vi "PC Main.vi"() -> ()   [LabVIEW 2021]
uses:
  Typedefs/Q FGV State Command.ctl
  Typedefs/Q Message Data.ctl
  <vilib>/event_ctls.llb/eventvkey.ctl
  <vilib>/Utility/error.llb/Error Cluster From Error Code.vi
  <vilib>/ErrorRing/Error Ring.xnode
panel:
  in  "Tab Control Application":enum32{"Home", "Measuring Panel"}(tab)
  in  "Connect Button":bool
  in  "NI-sbRIO-9651 IP address":string="10.8.5.60"
  in  "New Measurement Button":bool
  in  "Contact Button 1":bool
  in  "Close Button 1":bool
  in  "System Information Button 1":bool
  in  "Contact Button 2":bool
  in  "Close Button 2":bool
  in  "System Information Button 2":bool
  in  "Tab Control sbRIO":enum32{"Page 1"}(tab)
  in  "Reset Button":bool
  in  "Disconnect Button":bool
  # "3-Phase Power Meter \non the NI9651 circuit"
  # "NI-sbRIO-9651 Control"
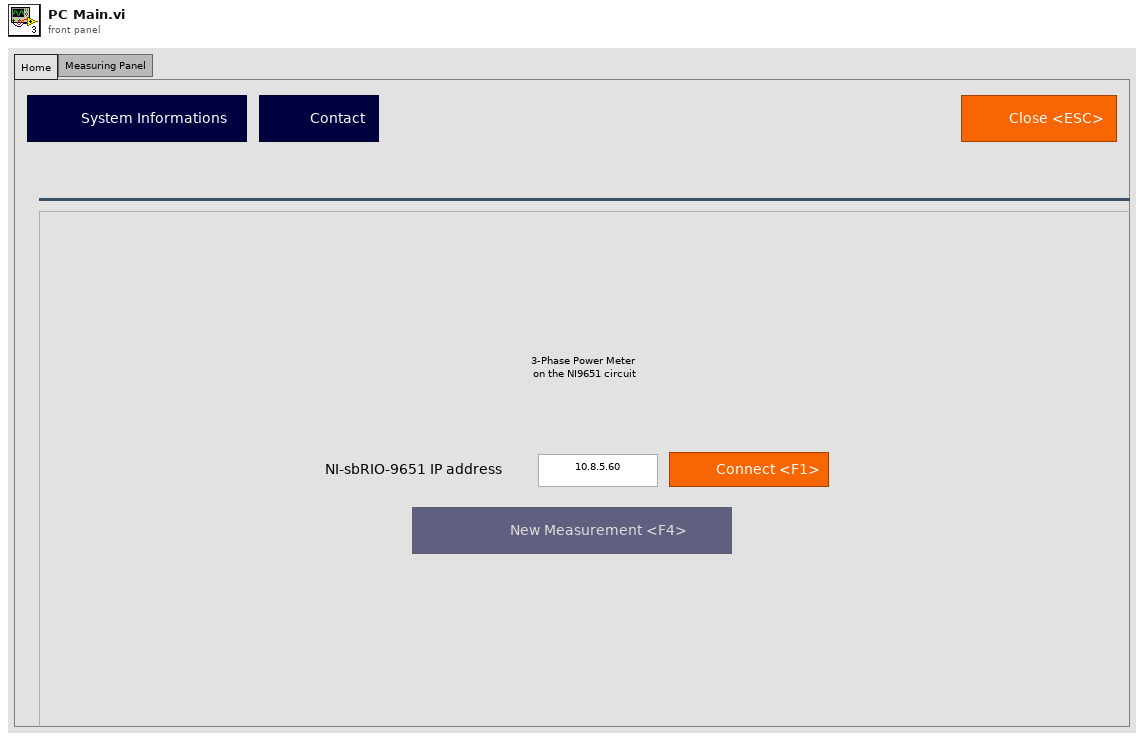
[diagram p1: front panel]
types:
  T1 = typedef "Q FGV State Command.ctl" = enum16{"Initialize", "Get", "Release"}
  T2 = typedef "Q Message Data.ctl" = cluster{"State Command":string, "Data":variant}
  T3 = enum8{"Enabled", "Disabled", "Disabled and Grayed Out"}
  T4 = typedef "eventvkey.ctl" = enum16{"ASCII", "Enter", "Return", "Shift", "Ctrl", "Alt", "Cmd", "Opt", "Caps", "NumLock", "Clear", "Break", "Up", "Down", "Left", "Right", "Insert", "Delete", "Home", "End", "PageUp", "PageDown", "Escape", "Help", "Pause", "ScrollLock", "F1", "F2", "F3", "F4", "F5", "F6", "F7", "F8", "F9", "F10", "F11", "F12", "F13", "F14", "F15", "F16", "F17", "F18", "F19", "F20", "F21", "F22", "F23", "F24", "Play", "VolumeUp", "VolumeDown", "Mute", "Two Byte Char"}
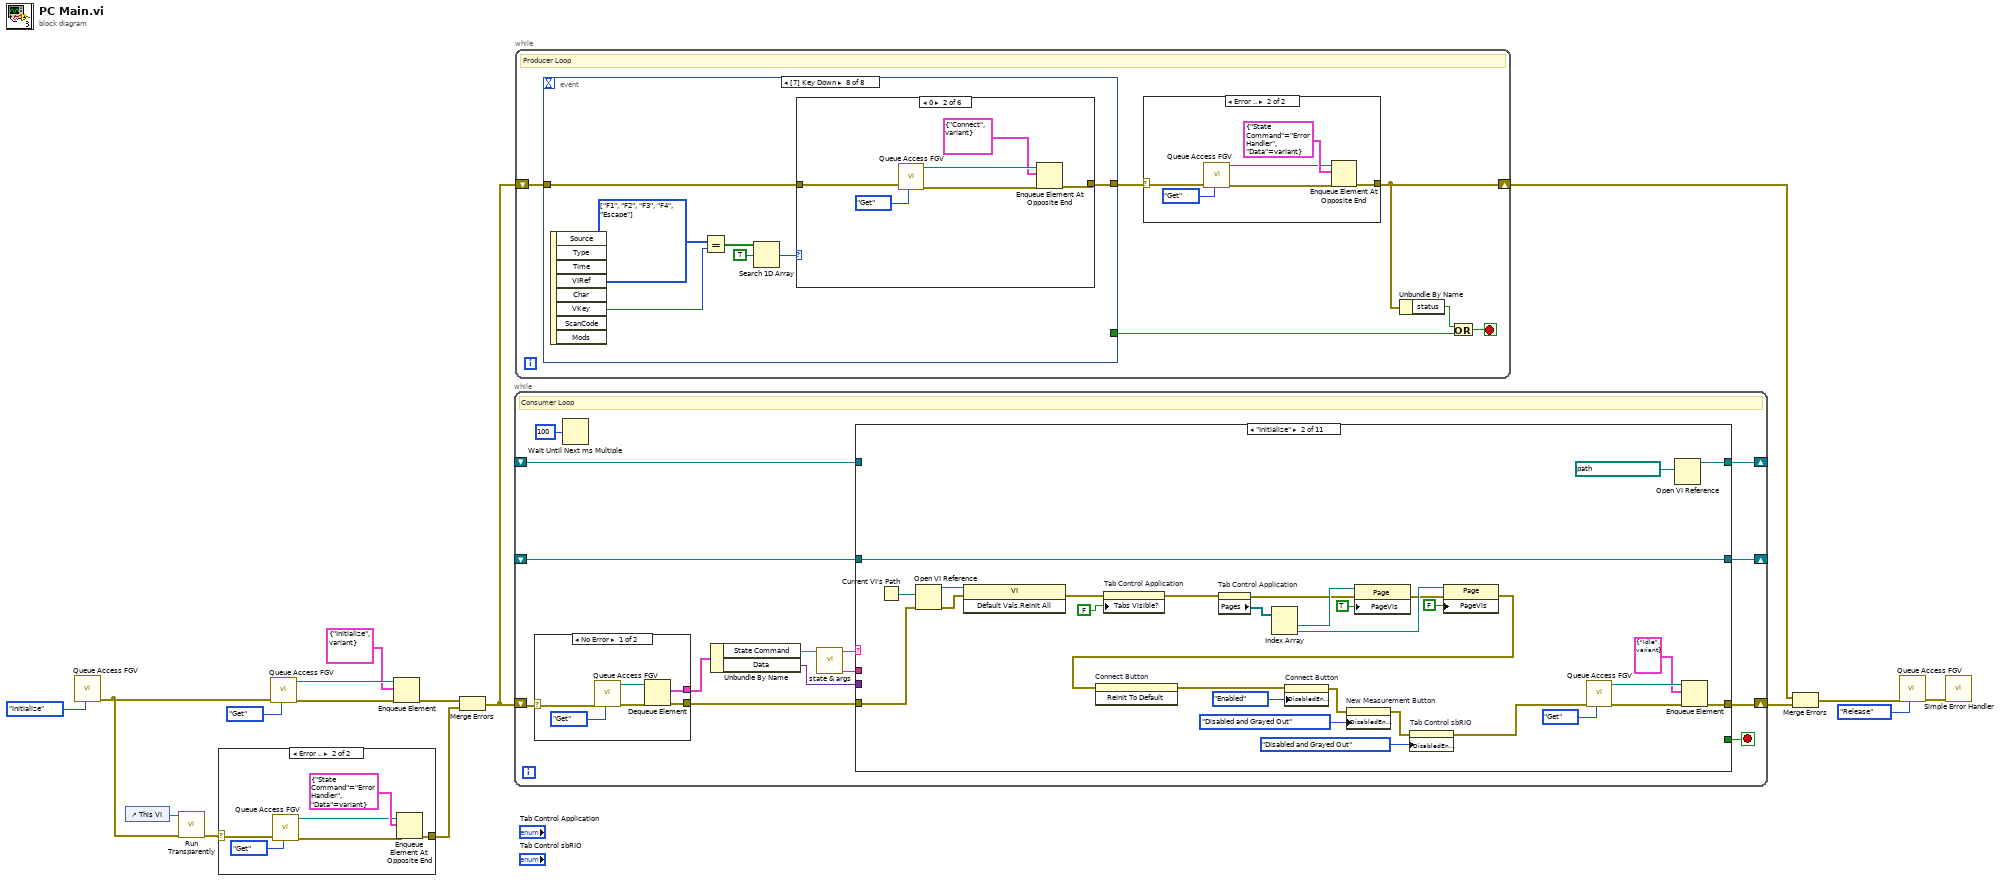
[diagram p0: block diagram]
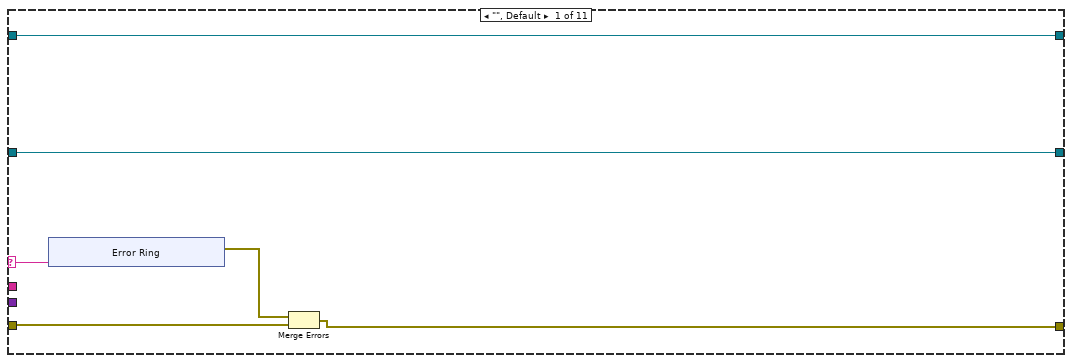
[diagram p3: hidden frame]
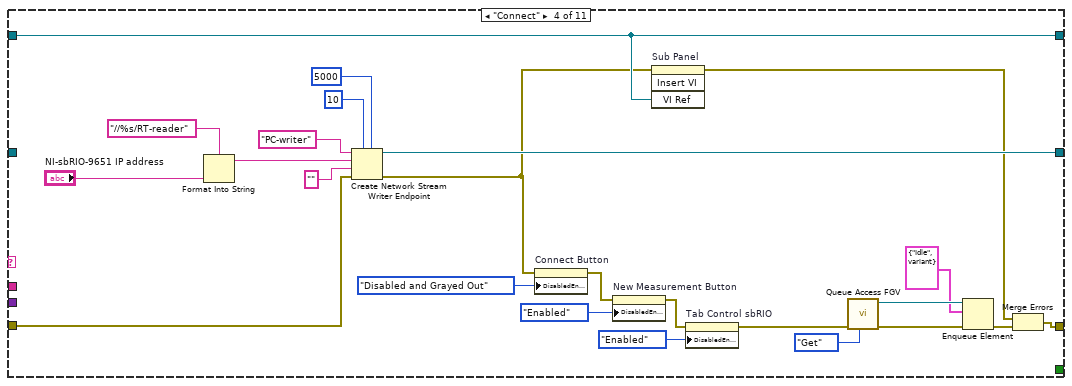
[diagram p5: hidden frame]
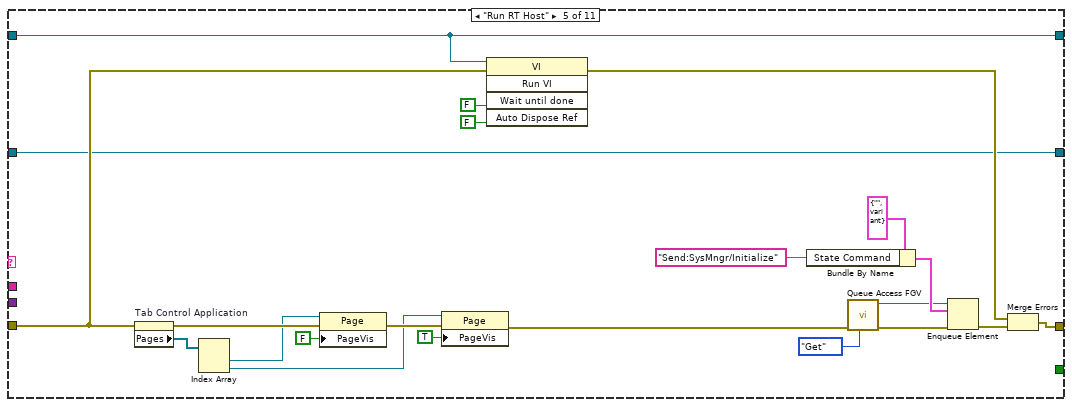
[diagram p6: hidden frame]
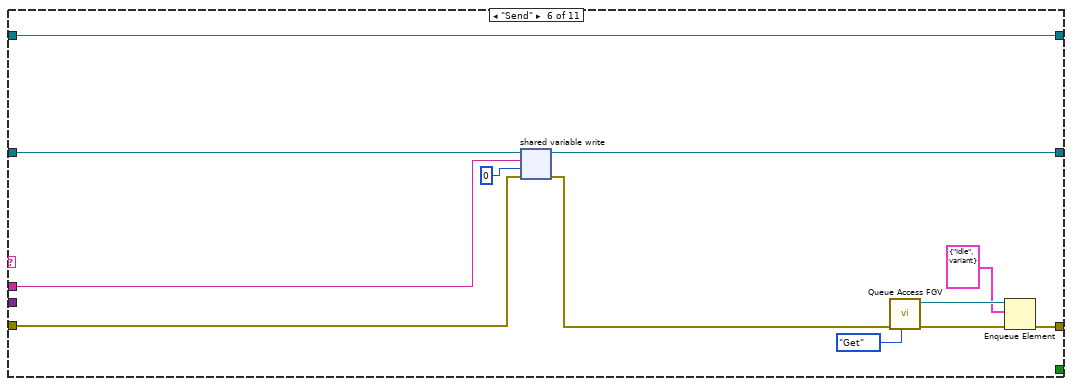
[diagram p7: hidden frame]
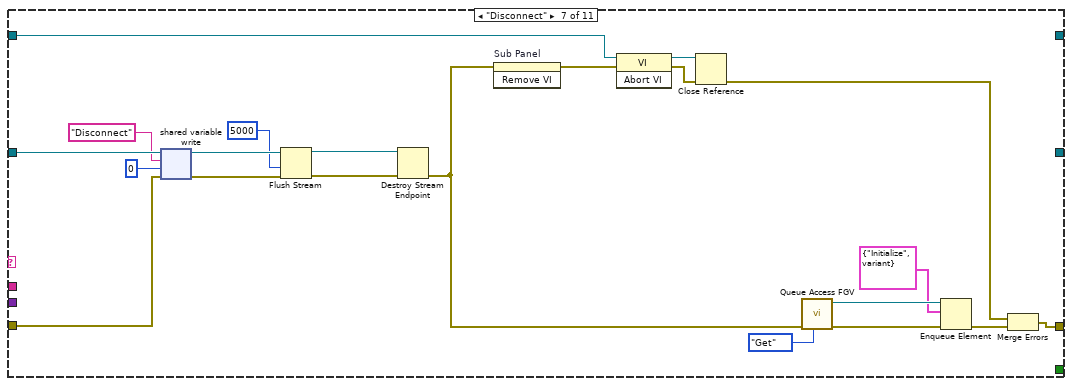
[diagram p8: hidden frame]
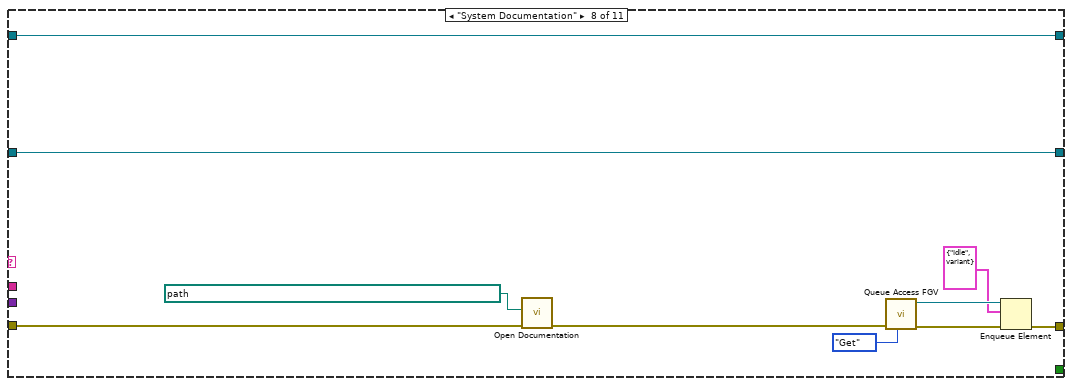
[diagram p9: hidden frame]
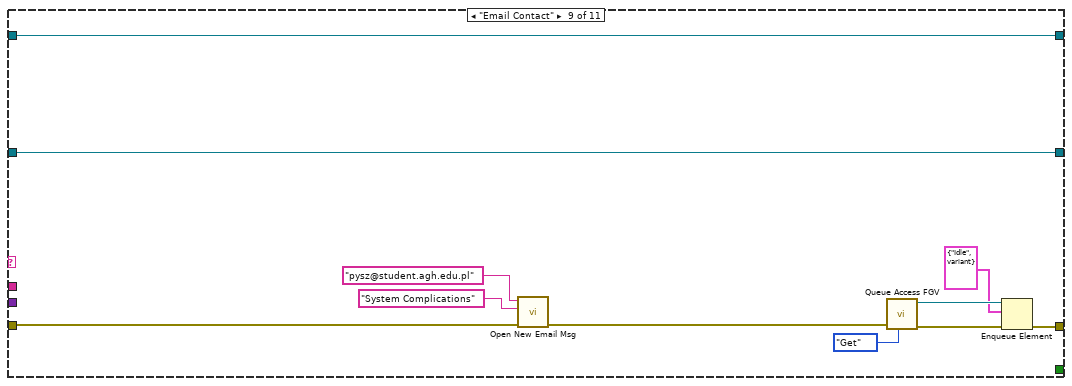
[diagram p10: hidden frame]
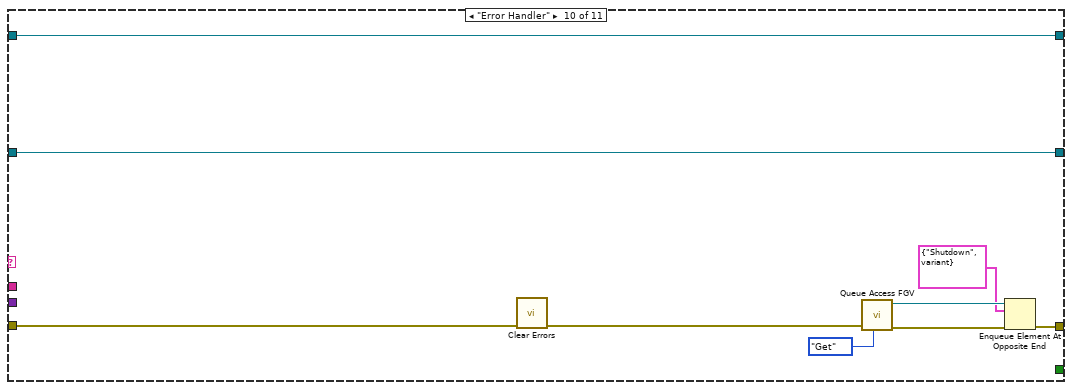
[diagram p11: hidden frame]
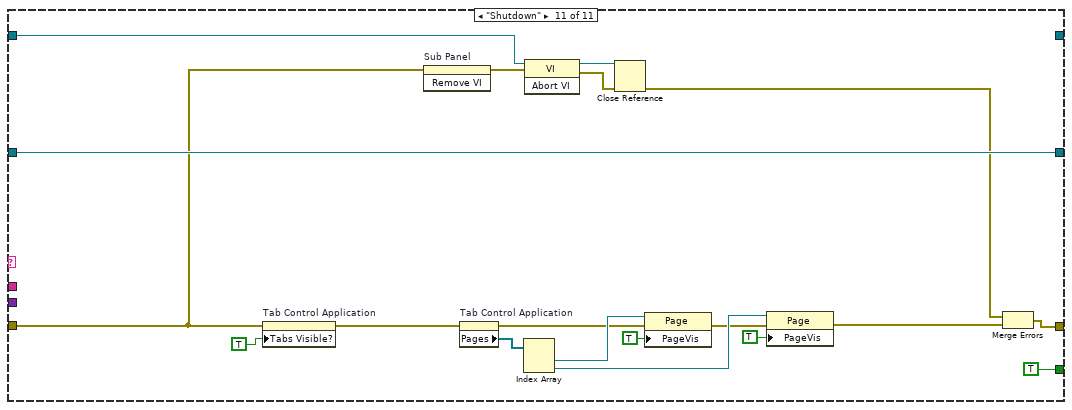
[diagram p12: hidden frame]
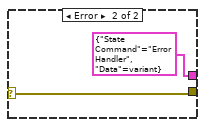
[diagram p13: hidden frame]
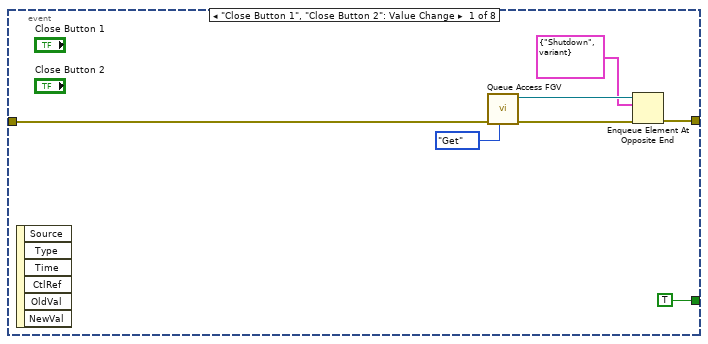
[diagram p14: hidden frame]
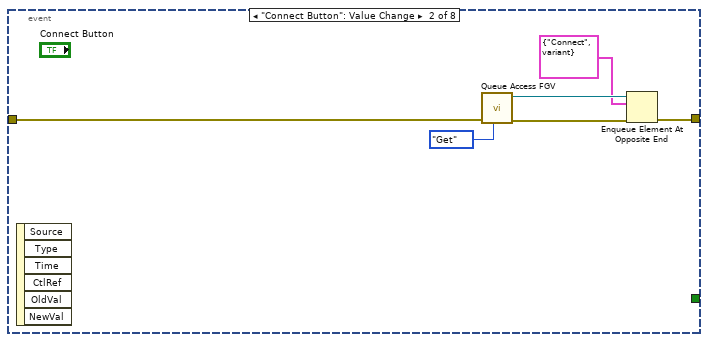
[diagram p15: hidden frame]
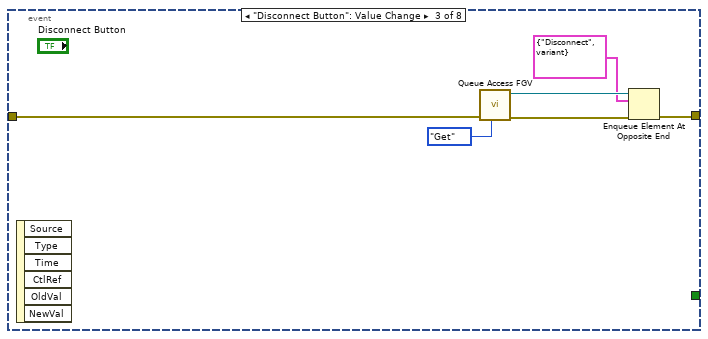
[diagram p16: hidden frame]
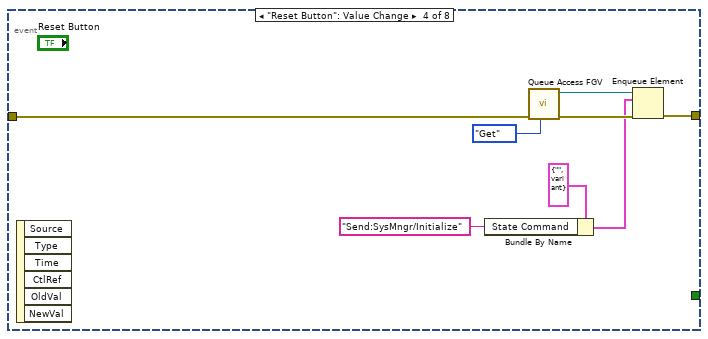
[diagram p17: hidden frame]
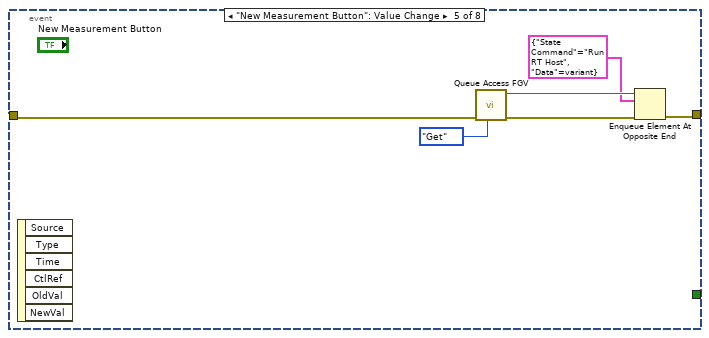
[diagram p18: hidden frame]
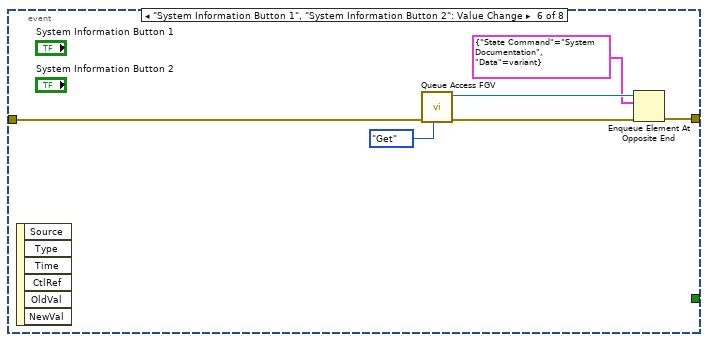
[diagram p19: hidden frame]
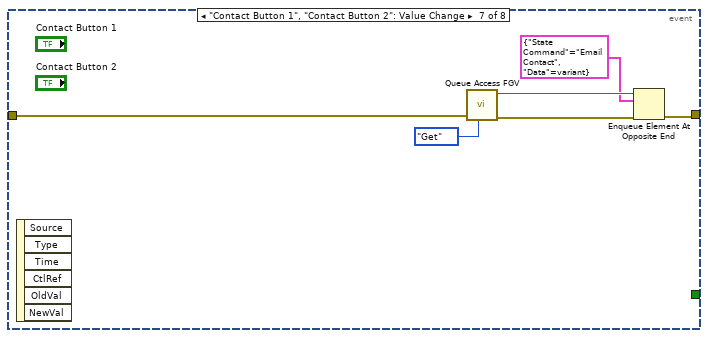
[diagram p20: hidden frame]
diagram:
  n1 = call "Queue Access FGV.vi"("FGV State Command"=Q_FGV_State_Command."Initialize") -> ("error out"=w5:errorcluster)  [unwired: 9 in, 1 out]
  n2 = control-ref of="This VI"() -> (w3:refnum<vi>)
  n3 = call "Run Transparently.vi"("error in (no error)"=w5, "This VI"=w3) -> ("error out"=w9:errorcluster)  [unwired: 9 in]
  n4 = case shown="Error .." w9 {
    selector: w9 -> [w17 w23]
    tunnel: [w17 w21] -> w6
    frame No Error {
    }
    frame Error {
      n5 = call "Queue Access FGV.vi"("FGV State Command"=Q_FGV_State_Command."Get", "error in (no error)"=w23) -> ("error out"=w22:errorcluster, "queue out"=w18:refnum<queue>)  [unwired: 8 in]
      n6 = Enqueue Element At Opposite End(queue=w18, element=T2 {"State Command"="Error Handler", "Data"=variant}, error in (no error)=w22) -> (error out=w21:errorcluster)  [unwired: 1 in, 2 out]
    }
  }
  n7 = call "Queue Access FGV.vi"("FGV State Command"=Q_FGV_State_Command."Get", "error in (no error)"=w5) -> ("error out"=w14:errorcluster, "queue out"=w15:refnum<queue>)  [unwired: 8 in]
  n8 = Enqueue Element(queue=w15, element=T2 {"State Command"="Initialize", "Data"=variant}, error in (no error)=w14) -> (error out=w7:errorcluster)  [unwired: 1 in, 2 out]
  n9 = Merge Errors(w7, w6) -> (w8:errorcluster)
  n10 = while {
    shift-right: [w27] -> _
    shift-left: _ -> [w28]
    shift-right: [w26] -> _
    shift-left: _ -> [w25]
    shift-right: [w24] -> w2
    shift-left: w8 -> [w37]
    stop <- w29 stop-if-true
    # "Consumer Loop"
    n11 = case shown="No Error" w37 {
      selector: w37 -> [w216 w219]
      tunnel: [w213 w219] -> w35
      tunnel: [w212 T2 {"State Command"="Error Handler", "Data"=variant} ("element")] -> w36
      frame No Error {
        n12 = call "Queue Access FGV.vi"("FGV State Command"=Q_FGV_State_Command."Get", "error in (no error)"=w216) -> ("error out"=w214:errorcluster, "queue out"=w217:refnum<queue>)  [unwired: 8 in]
        n13 = Dequeue Element(queue=w217, error in (no error)=w214) -> (element=w212:T2, error out=w213:errorcluster)  [unwired: 1 in, 2 out]
      }
      frame Error {
      }
    }
    n14 = Wait Until Next ms Multiple(millisecond multiple=u32 100) -> ()  [unwired: 1 out]
    n15 = Unbundle By Name(w36) -> ("State Command"=w34:string, "Data"=w31:variant)
    n16 = call "state & args.vi"("state:args"=w34) -> ("args"=w32:string, "state"=w33:string)  [unwired: 9 in]
    n17 = case shown="\"Initialize\"" w33 {
      selector: w33 -> [w43 _ _ _ _ _ _ _ _ _ _]
      tunnel: w35 -> [w41 w67 w83 w88 w112 w141 w155 w167 w178 w192 w196]
      tunnel: [w40 w73 w83 w85 w110 w133 w143 w168 w179 w186 w194] -> w24
      tunnel: w32 -> [_ _ _ _ _ w138 _ _ _ _ _]
      tunnel: w31 -> [_ _ _ _ _ _ _ _ _ _ _]
      tunnel: [_ _ _ _ _ _ _ _ _ _ TRUE] -> w29
      tunnel: w28 -> [w39 w51 w82 _ w108 w140 w158 w164 w173 w185 w210]
      tunnel: [w39 w51 w82 w94 w108 w139 _ w164 w173 w185 w210] -> w27
      tunnel: [w38 w52 w81 w89 w113 w131 _ w163 w174 w184 _] -> w26
      tunnel: w25 -> [w38 _ w81 w89 w113 w131 w148 w163 w174 w184 w200]
      frame "", Default {
        n18 = xnode "Error Ring"("parameter 0"=w43) -> ("error out"=w42:errorcluster)
        n19 = Merge Errors(w42, w41) -> (w40:errorcluster)
      }
      frame "Initialize" {
        n20 = Current VI's Path() -> (path=w80:path)
        n21 = Open VI Reference(vi path=w80, error in (no error)=w67) -> (vi reference=w79:refnum<vi>, error out=w78:errorcluster)  [unwired: 4 in]
        n22 = invoke class="VI" method="Default Vals.Reinit All"(reference=w79, error in=w78) -> (error out=w57:errorcluster)  [unwired: 1 in, 2 out]
        n23 = property on="Tab Control Application" class="TabCtl (strict)"(error in=w57, "Tabs Visible?"=FALSE) -> (error out=w66:errorcluster)  [unwired: 1 in, 1 out]
        n24 = property on="Tab Control Application" class="TabCtl (strict)"(error in=w66) -> (error out=w62:errorcluster, "Pages"=w61:refnum<vi>[])  [unwired: 1 in, 1 out]
        n25 = Index Array(array=w61) -> (element #1=w63:refnum<vi>, element #2=w65:refnum<vi>)  [unwired: 2 in]
        n26 = property class="Page"(reference=w63, error in=w62, "PageVis"=TRUE ("Page Visible")) -> (error out=w64:errorcluster)  [unwired: 1 out]
        n27 = property class="Page"(reference=w65, error in=w64, "PageVis"=FALSE ("Page Visible")) -> (error out=w55:errorcluster)  [unwired: 1 out]
        n28 = invoke on="Connect Button" class="Bool" method="Reinit To Default"(error in=w55) -> (error out=w56:errorcluster)  [unwired: 2 in, 2 out]
        n29 = property on="Connect Button" class="Bool"(error in=w56, "DisabledEnum"=T3."Enabled" ("Disabled")) -> (error out=w54:errorcluster)  [unwired: 1 in, 1 out]
        n30 = property on="New Measurement Button" class="Bool"(error in=w54, "DisabledEnum"=T3."Disabled and Grayed Out" ("Disabled")) -> (error out=w70:errorcluster)  [unwired: 1 in, 1 out]
        n31 = property on="Tab Control sbRIO" class="TabCtl (strict)"(error in=w70, "DisabledEnum"=T3."Disabled and Grayed Out" ("Disabled")) -> (error out=w69:errorcluster)  [unwired: 1 in, 1 out]
        n32 = call "Queue Access FGV.vi"("FGV State Command"=Q_FGV_State_Command."Get", "error in (no error)"=w69) -> ("error out"=w75:errorcluster, "queue out"=w76:refnum<queue>)  [unwired: 8 in]
        n33 = Open VI Reference(vi path=path "F:/AGH - Inżynieria Biomedyczna (I i II stopień)/PRACA MAGISTERSKA/FPGA Project - POWER METER/RT Host/RT Main.vi") -> (vi reference=w52:refnum<vi>)  [unwired: 5 in, 1 out]
        n34 = Enqueue Element(queue=w76, element=T2 {"State Command"="Idle", "Data"=variant}, error in (no error)=w75) -> (error out=w73:errorcluster)  [unwired: 1 in, 2 out]
      }
      frame "Idle" {
      }
      frame "Connect" {
        n35 = Format Into String(format string="//%s/RT-reader", "NI-sbRIO-9651 IP address") -> (resulting string=w99:string)  [unwired: 2 in, 1 out]
        n36 = Create Network Stream Writer Endpoint(5:5000 ("timeout in ms (-1)"), 7:10 ("writer buffer size"), 8:w88, 9:"", 10:w99, 11:"PC-writer" ("writer name")) -> (0:w87:errorcluster, 3:w94:refnum<k21>)  [unwired: 1 in]
        n37 = property on="Connect Button" class="Bool"(error in=w87, "DisabledEnum"=T3."Disabled and Grayed Out" ("Disabled")) -> (error out=w92:errorcluster)  [unwired: 1 in, 1 out]
        n38 = property on="New Measurement Button" class="Bool"(error in=w92, "DisabledEnum"=T3."Enabled" ("Disabled")) -> (error out=w90:errorcluster)  [unwired: 1 in, 1 out]
        n39 = invoke on="Sub Panel" class="SubPanel" method="Insert VI"(error in=w87, "VI Ref"=w89) -> (error out=w84:errorcluster)  [unwired: 2 in, 3 out]
        n40 = property on="Tab Control sbRIO" class="TabCtl (strict)"(error in=w90, "DisabledEnum"=T3."Enabled" ("Disabled")) -> (error out=w93:errorcluster)  [unwired: 1 in, 1 out]
        n41 = call "Queue Access FGV.vi"("FGV State Command"=Q_FGV_State_Command."Get", "error in (no error)"=w93) -> ("error out"=w105:errorcluster, "queue out"=w106:refnum<queue>)  [unwired: 8 in]
        n42 = Enqueue Element(queue=w106, element=T2 {"State Command"="Idle", "Data"=variant}, error in (no error)=w105) -> (error out=w86:errorcluster)  [unwired: 1 in, 2 out]
        n43 = Merge Errors(w84, w86) -> (w85:errorcluster)
      }
      frame "Run RT Host" {
        n44 = property on="Tab Control Application" class="TabCtl (strict)"(error in=w112) -> (error out=w126:errorcluster, "Pages"=w127:refnum<vi>[])  [unwired: 1 in, 1 out]
        n45 = Index Array(array=w127) -> (element #1=w125:refnum<vi>, element #2=w123:refnum<vi>)  [unwired: 2 in]
        n46 = property class="Page"(reference=w125, error in=w126, "PageVis"=FALSE ("Page Visible")) -> (error out=w124:errorcluster)  [unwired: 1 out]
        n47 = property class="Page"(reference=w123, error in=w124, "PageVis"=TRUE ("Page Visible")) -> (error out=w129:errorcluster)  [unwired: 1 out]
        n48 = invoke class="VI" method="Run VI"(reference=w113, error in=w112, "Wait until done"=FALSE ("Wait Until Done"), "Auto Dispose Ref"=FALSE ("Auto Dispose Reference")) -> (error out=w109:errorcluster)  [unwired: 1 in, 4 out]
        n49 = Bundle By Name(cluster=T2 {"State Command"="", "Data"=variant} ("element"), "State Command"="Send:SysMngr/Initialize") -> (w120:T2)
        n50 = call "Queue Access FGV.vi"("FGV State Command"=Q_FGV_State_Command."Get", "error in (no error)"=w129) -> ("error out"=w117:errorcluster, "queue out"=w118:refnum<queue>)  [unwired: 8 in]
        n51 = Enqueue Element(queue=w118, element=w120, error in (no error)=w117) -> (error out=w111:errorcluster)  [unwired: 1 in, 2 out]
        n52 = Merge Errors(w109, w111) -> (w110:errorcluster)
      }
      frame "Send" {
        n53 = shared-variable-write(w140, w141, w138, 0 ("timeout ms (-1)")) -> (w139:refnum<k21>, w132:errorcluster)  [unwired: 1 out]
        n54 = call "Queue Access FGV.vi"("FGV State Command"=Q_FGV_State_Command."Get", "error in (no error)"=w132) -> ("error out"=w134:errorcluster, "queue out"=w135:refnum<queue>)  [unwired: 8 in]
        n55 = Enqueue Element(queue=w135, element=T2 {"State Command"="Idle", "Data"=variant}, error in (no error)=w134) -> (error out=w133:errorcluster)  [unwired: 1 in, 2 out]
      }
      frame "Disconnect" {
        n56 = shared-variable-write(w158, w155, "Disconnect" ("data in"), 0 ("timeout ms (-1)")) -> (w154:refnum<k21>, w153:errorcluster)  [unwired: 1 out]
        n57 = Flush Stream(8:w153, 9:5000 ("timeout in ms (-1)"), 11:w154) -> (0:w150:errorcluster, 3:w151:refnum<k21>)  [unwired: 1 in, 1 out]
        n58 = Destroy Stream Endpoint(8:w150, 11:w151) -> (0:w147:errorcluster)
        n59 = invoke on="Sub Panel" class="SubPnl" method="Remove VI"(error in=w147) -> (error out=w149:errorcluster)  [unwired: 2 in, 2 out]
        n60 = invoke class="VI" method="Abort VI"(reference=w148, error in=w149) -> (reference out=w146:refnum<vi>, error out=w145:errorcluster)  [unwired: 1 in, 1 out]
        n61 = Close Reference(reference=w146, error in (no error)=w145) -> (error out=w142:errorcluster)
        n62 = call "Queue Access FGV.vi"("FGV State Command"=Q_FGV_State_Command."Get", "error in (no error)"=w147) -> ("error out"=w160:errorcluster, "queue out"=w161:refnum<queue>)  [unwired: 8 in]
        n63 = Enqueue Element(queue=w161, element=T2 {"State Command"="Initialize", "Data"=variant}, error in (no error)=w160) -> (error out=w144:errorcluster)  [unwired: 1 in, 2 out]
        n64 = Merge Errors(w142, w144) -> (w143:errorcluster)
      }
      frame "System Documentation" {
        n65 = call "Open Documentation.vi"("error in (no error)"=w167, "File Path"=path "/\"F/AGH - Inżynieria Biomedyczna (I i II stopień)/PRACA MAGISTERSKA/FPGA Project - POWER METER/DOKUMENTACJA.pdf\"") -> ("error out"=w166:errorcluster)  [unwired: 9 in]
        n66 = call "Queue Access FGV.vi"("FGV State Command"=Q_FGV_State_Command."Get", "error in (no error)"=w166) -> ("error out"=w170:errorcluster, "queue out"=w171:refnum<queue>)  [unwired: 8 in]
        n67 = Enqueue Element(queue=w171, element=T2 {"State Command"="Idle", "Data"=variant}, error in (no error)=w170) -> (error out=w168:errorcluster)  [unwired: 1 in, 2 out]
      }
      frame "Email Contact" {
        n68 = call "Open New Email Msg.vi"("error in (no error)"=w178, "Subject"="System Complications", "Recipient"="pysz@student.agh.edu.pl") -> ("error out"=w177:errorcluster)  [unwired: 8 in]
        n69 = call "Queue Access FGV.vi"("FGV State Command"=Q_FGV_State_Command."Get", "error in (no error)"=w177) -> ("error out"=w181:errorcluster, "queue out"=w182:refnum<queue>)  [unwired: 8 in]
        n70 = Enqueue Element(queue=w182, element=T2 {"State Command"="Idle", "Data"=variant}, error in (no error)=w181) -> (error out=w179:errorcluster)  [unwired: 1 in, 2 out]
      }
      frame "Error Handler" {
        n71 = call <vilib>:"Clear Errors.vi"("error in (no error)"=w192) -> ("error out"=w187:errorcluster)  [unwired: 5 in, 1 out]
        n72 = call "Queue Access FGV.vi"("FGV State Command"=Q_FGV_State_Command."Get", "error in (no error)"=w187) -> ("error out"=w190:errorcluster, "queue out"=w189:refnum<queue>)  [unwired: 8 in]
        n73 = Enqueue Element At Opposite End(queue=w189, element=T2 {"State Command"="Shutdown", "Data"=variant}, error in (no error)=w190) -> (error out=w186:errorcluster)  [unwired: 1 in, 2 out]
      }
      frame "Shutdown" {
        n74 = property on="Tab Control Application" class="TabCtl (strict)"(error in=w196, "Tabs Visible?"=TRUE) -> (error out=w202:errorcluster)  [unwired: 1 in, 1 out]
        n75 = invoke on="Sub Panel" class="SubPnl" method="Remove VI"(error in=w196) -> (error out=w199:errorcluster)  [unwired: 2 in, 2 out]
        n76 = property on="Tab Control Application" class="TabCtl (strict)"(error in=w202) -> (error out=w204:errorcluster, "Pages"=w203:refnum<vi>[])  [unwired: 1 in, 1 out]
        n77 = Index Array(array=w203) -> (element #1=w205:refnum<vi>, element #2=w207:refnum<vi>)  [unwired: 2 in]
        n78 = invoke class="VI" method="Abort VI"(reference=w200, error in=w199) -> (reference out=w198:refnum<vi>, error out=w197:errorcluster)  [unwired: 1 in, 1 out]
        n79 = Close Reference(reference=w198, error in (no error)=w197) -> (error out=w193:errorcluster)
        n80 = property class="Page"(reference=w205, error in=w204, "PageVis"=TRUE ("Page Visible")) -> (error out=w206:errorcluster)  [unwired: 1 out]
        n81 = property class="Page"(reference=w207, error in=w206, "PageVis"=TRUE ("Page Visible")) -> (error out=w195:errorcluster)  [unwired: 1 out]
        n82 = Merge Errors(w193, w195) -> (w194:errorcluster)
      }
    }
  }
  n83 = while {
    shift-right: [w220] -> w1
    shift-left: w8 -> [w223]
    stop <- w225 stop-if-true
    # "Producer Loop"
    n84 = event shown="[7] Key Down" {
      selector: _ -> [_ _ _ _ _ _ _ _]
      dyn-events: _ -> [_ _ _ _ _ _ _ _]
      timeout: _ -> [_ _ _ _ _ _ _ _]
      tunnel: w223 -> [w232 w233 w239 w246 w253 w259 w265 w272]
      tunnel: [w229 w234 w240 w247 w254 w260 w266 w271] -> w222
      tunnel: [TRUE _ _ _ _ _ _ _] -> w221
      event "Close Button 1", "Close Button 2": Value Change {
        n85 = event-data() -> ()  [unwired: 1 in, 6 out]
        n86 = call "Queue Access FGV.vi"("FGV State Command"=Q_FGV_State_Command."Get", "error in (no error)"=w232) -> ("error out"=w230:errorcluster, "queue out"=w228:refnum<queue>)  [unwired: 8 in]
        n87 = Enqueue Element At Opposite End(queue=w228, element=T2 {"State Command"="Shutdown", "Data"=variant}, error in (no error)=w230) -> (error out=w229:errorcluster)  [unwired: 1 in, 2 out]
      }
      event "Connect Button": Value Change {
        n88 = event-data() -> ()  [unwired: 1 in, 6 out]
        n89 = call "Queue Access FGV.vi"("FGV State Command"=Q_FGV_State_Command."Get", "error in (no error)"=w233) -> ("error out"=w237:errorcluster, "queue out"=w236:refnum<queue>)  [unwired: 8 in]
        n90 = Enqueue Element At Opposite End(queue=w236, element=T2 {"State Command"="Connect", "Data"=variant}, error in (no error)=w237) -> (error out=w234:errorcluster)  [unwired: 1 in, 2 out]
      }
      event "Disconnect Button": Value Change {
        n91 = event-data() -> ()  [unwired: 1 in, 6 out]
        n92 = call "Queue Access FGV.vi"("FGV State Command"=Q_FGV_State_Command."Get", "error in (no error)"=w239) -> ("error out"=w243:errorcluster, "queue out"=w242:refnum<queue>)  [unwired: 8 in]
        n93 = Enqueue Element At Opposite End(queue=w242, element=T2 {"State Command"="Disconnect", "Data"=variant}, error in (no error)=w243) -> (error out=w240:errorcluster)  [unwired: 1 in, 2 out]
      }
      event "Reset Button": Value Change {
        n94 = event-data() -> ()  [unwired: 1 in, 6 out]
        n95 = Bundle By Name(cluster=T2 {"State Command"="", "Data"=variant} ("element"), "State Command"="Send:SysMngr/Initialize") -> (w248:T2)
        n96 = call "Queue Access FGV.vi"("FGV State Command"=Q_FGV_State_Command."Get", "error in (no error)"=w246) -> ("error out"=w251:errorcluster, "queue out"=w250:refnum<queue>)  [unwired: 8 in]
        n97 = Enqueue Element(queue=w250, element=w248, error in (no error)=w251) -> (error out=w247:errorcluster)  [unwired: 1 in, 2 out]
      }
      event "New Measurement Button": Value Change {
        n98 = event-data() -> ()  [unwired: 1 in, 6 out]
        n99 = call "Queue Access FGV.vi"("FGV State Command"=Q_FGV_State_Command."Get", "error in (no error)"=w253) -> ("error out"=w257:errorcluster, "queue out"=w256:refnum<queue>)  [unwired: 8 in]
        n100 = Enqueue Element At Opposite End(queue=w256, element=T2 {"State Command"="Run RT Host", "Data"=variant}, error in (no error)=w257) -> (error out=w254:errorcluster)  [unwired: 1 in, 2 out]
      }
      event "System Information Button 1", "System Information Button 2": Value Change {
        n101 = event-data() -> ()  [unwired: 1 in, 6 out]
        n102 = call "Queue Access FGV.vi"("FGV State Command"=Q_FGV_State_Command."Get", "error in (no error)"=w259) -> ("error out"=w263:errorcluster, "queue out"=w262:refnum<queue>)  [unwired: 8 in]
        n103 = Enqueue Element At Opposite End(queue=w262, element=T2 {"State Command"="System Documentation", "Data"=variant}, error in (no error)=w263) -> (error out=w260:errorcluster)  [unwired: 1 in, 2 out]
      }
      event "Contact Button 1", "Contact Button 2": Value Change {
        n104 = event-data() -> ()  [unwired: 1 in, 6 out]
        n105 = call "Queue Access FGV.vi"("FGV State Command"=Q_FGV_State_Command."Get", "error in (no error)"=w265) -> ("error out"=w269:errorcluster, "queue out"=w268:refnum<queue>)  [unwired: 8 in]
        n106 = Enqueue Element At Opposite End(queue=w268, element=T2 {"State Command"="Email Contact", "Data"=variant}, error in (no error)=w269) -> (error out=w266:errorcluster)  [unwired: 1 in, 2 out]
      }
      event Key Down {
        w277 = T4[] [enum."F1", enum."F2", enum."F3", enum."F4", enum."Escape"] items=["ASCII", "Enter", "Return", "Shift", "Ctrl", "Alt", "Cmd", "Opt", "Caps", "NumLock", "Clear", "Break", "Up", "Down", "Left", "Right", "Insert", "Delete", "Home", "End", "PageUp", "PageDown", "Escape", "Help", "Pause", "ScrollLock", "F1", "F2", "F3", "F4", "F5", "F6", "F7", "F8", "F9", "F10", "F11", "F12", "F13", "F14", "F15", "F16", "F17", "F18", "F19", "F20", "F21", "F22", "F23", "F24", "Play", "VolumeUp", "VolumeDown", "Mute", "Two Byte Char"]
        n107 = event-data() -> ("VKey"=w276:T4)  [unwired: 1 in, 7 out]
        n108 = Equal?(x=w277, y=w276) -> (x = y?=w275:bool[])
        n109 = Search 1D Array(1D array=w275, element=TRUE) -> (index of element=w273:i32)  [unwired: 1 in]
        n110 = case shown="0" w273 {
          tunnel: w272 -> [w279 w285 w291 w299 w305 w311]
          tunnel: [w278 w284 w290 w298 w304 w310] -> w271
          frame Default {
            n111 = call "Queue Access FGV.vi"("FGV State Command"=Q_FGV_State_Command."Get", "error in (no error)"=w279) -> ("error out"=w282:errorcluster, "queue out"=w281:refnum<queue>)  [unwired: 8 in]
            n112 = Enqueue Element At Opposite End(queue=w281, element=T2 {"State Command"="Idle", "Data"=variant}, error in (no error)=w282) -> (error out=w278:errorcluster)  [unwired: 1 in, 2 out]
          }
          frame 0 {
            n113 = call "Queue Access FGV.vi"("FGV State Command"=Q_FGV_State_Command."Get", "error in (no error)"=w285) -> ("error out"=w288:errorcluster, "queue out"=w287:refnum<queue>)  [unwired: 8 in]
            n114 = Enqueue Element At Opposite End(queue=w287, element=T2 {"State Command"="Connect", "Data"=variant}, error in (no error)=w288) -> (error out=w284:errorcluster)  [unwired: 1 in, 2 out]
          }
          frame 1 {
            n115 = Bundle By Name(cluster=T2 {"State Command"="", "Data"=variant} ("element"), "State Command"="Send:SysMngr/Initialize") -> (w293:T2)
            n116 = call "Queue Access FGV.vi"("FGV State Command"=Q_FGV_State_Command."Get", "error in (no error)"=w291) -> ("error out"=w296:errorcluster, "queue out"=w295:refnum<queue>)  [unwired: 8 in]
            n117 = Enqueue Element(queue=w295, element=w293, error in (no error)=w296) -> (error out=w290:errorcluster)  [unwired: 1 in, 2 out]
          }
          frame 2 {
            n118 = call "Queue Access FGV.vi"("FGV State Command"=Q_FGV_State_Command."Get", "error in (no error)"=w299) -> ("error out"=w302:errorcluster, "queue out"=w301:refnum<queue>)  [unwired: 8 in]
            n119 = Enqueue Element At Opposite End(queue=w301, element=T2 {"State Command"="Disconnect", "Data"=variant}, error in (no error)=w302) -> (error out=w298:errorcluster)  [unwired: 1 in, 2 out]
          }
          frame 3 {
            n120 = call "Queue Access FGV.vi"("FGV State Command"=Q_FGV_State_Command."Get", "error in (no error)"=w305) -> ("error out"=w308:errorcluster, "queue out"=w307:refnum<queue>)  [unwired: 8 in]
            n121 = Enqueue Element At Opposite End(queue=w307, element=T2 {"State Command"="New Measurement", "Data"=variant}, error in (no error)=w308) -> (error out=w304:errorcluster)  [unwired: 1 in, 2 out]
          }
          frame 4 {
            n122 = call "Queue Access FGV.vi"("FGV State Command"=Q_FGV_State_Command."Get", "error in (no error)"=w311) -> ("error out"=w314:errorcluster, "queue out"=w313:refnum<queue>)  [unwired: 8 in]
            n123 = Enqueue Element At Opposite End(queue=w313, element=T2 {"State Command"="Shutdown", "Data"=variant}, error in (no error)=w314) -> (error out=w310:errorcluster)  [unwired: 1 in, 2 out]
          }
        }
      }
    }
    n124 = case shown="Error .." w222 {
      selector: w222 -> [w316 w322]
      tunnel: [w316 w320] -> w220
      frame No Error {
      }
      frame Error {
        n125 = call "Queue Access FGV.vi"("FGV State Command"=Q_FGV_State_Command."Get", "error in (no error)"=w322) -> ("error out"=w321:errorcluster, "queue out"=w317:refnum<queue>)  [unwired: 8 in]
        n126 = Enqueue Element At Opposite End(queue=w317, element=T2 {"State Command"="Error Handler", "Data"=variant}, error in (no error)=w321) -> (error out=w320:errorcluster)  [unwired: 1 in, 2 out]
      }
    }
    n127 = Unbundle By Name(w220) -> ("status"=w224:bool)
    n128 = Or(x=w224, y=w221) -> (x .or. y?=w225:bool)
  }
  n129 = Merge Errors(w1, w2) -> (w10:errorcluster)
  n130 = call "Queue Access FGV.vi"("FGV State Command"=Q_FGV_State_Command."Release", "error in (no error)"=w10) -> ("error out"=w11:errorcluster)  [unwired: 8 in, 1 out]
  n131 = call <vilib>:"Simple Error Handler.vi"("error in (no error)"=w11) -> ()  [unwired: 4 in, 5 out]
